vi "ZMQ sandbox.vi"() -> ()   [LabVIEW 2019]
uses:
  <vilib>/addons/zeromq/zmq_context.lvclass
  <vilib>/addons/zeromq/zmq_socket.lvclass
  <vilib>/addons/zeromq/socket_type.ctl
  <vilib>/addons/zeromq/zeromq.lvlib
  <vilib>/addons/_JKI Toolkits/Caraya/classes/Test/Test.lvclass
panel:
  in  "stop":bool
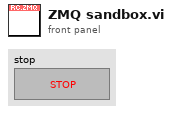
[diagram p1: front panel]
types:
  T1 = typedef "zeromq.lvlib/socket_type.ctl" = enum8{"ZMQ_PAIR", "ZMQ_PUB", "ZMQ_SUB", "ZMQ_REQ", "ZMQ_REP", "ZMQ_DEALER", "ZMQ_ROUTER", "ZMQ_PULL", "ZMQ_PUSH", "ZMQ_XPUB", "ZMQ_XSUB", "ZMQ_STREAM", "ZMQ_SERVER", "ZMQ_CLIENT", "ZMQ_RADIO", "ZMQ_DISH", "ZMQ_GATHER", "ZMQ_SCATTER", "ZMQ_DGRAM"}
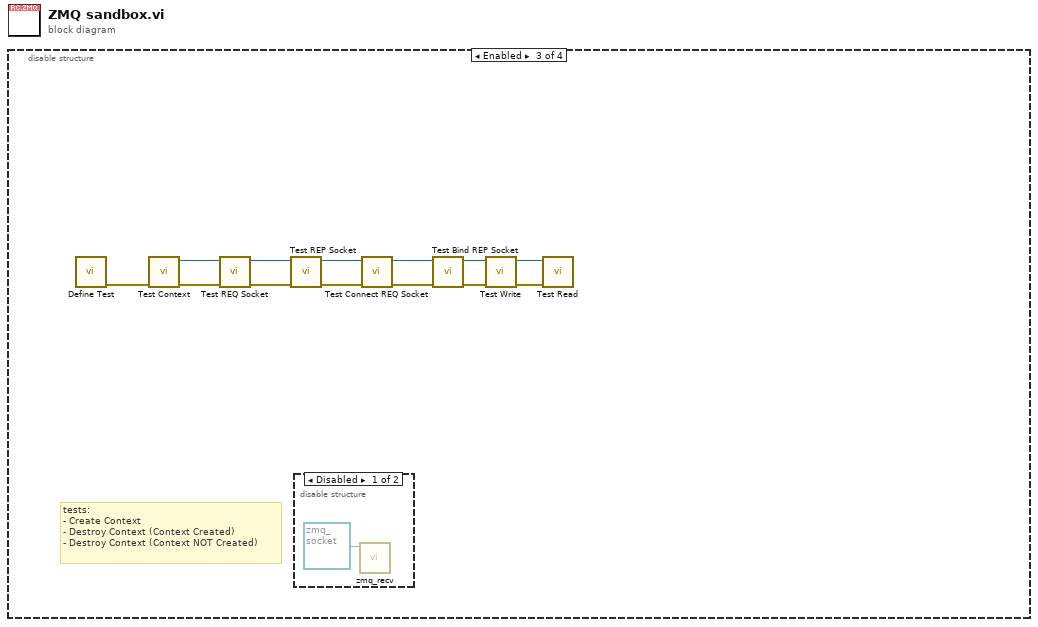
[diagram p0: block diagram]
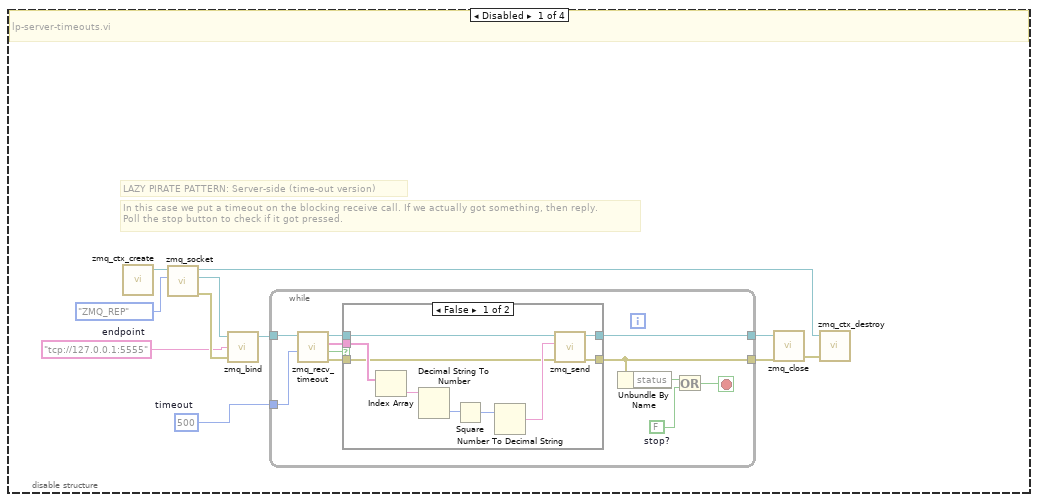
[diagram p2: hidden frame]
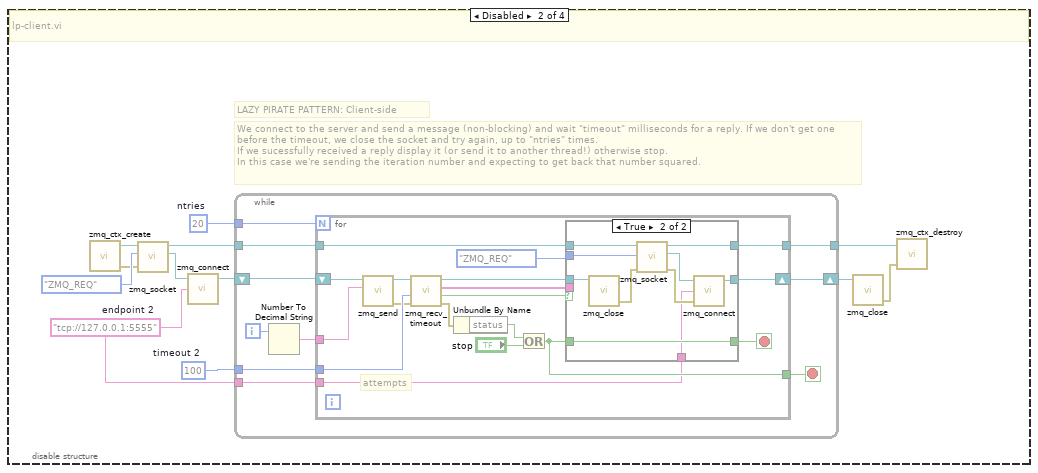
[diagram p4: hidden frame]
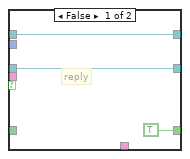
[diagram p5: hidden frame]
diagram:
  n1 = disable-structure "Diagram Disable Structure" shown="Enabled" {
    frame Disabled {
      w11 = u32 500  # timeout
      w9 = "tcp://127.0.0.1:5555"  # endpoint
      # "In this case we put a timeout on the blocking receive call. If we actually got something, then reply.\nPoll the stop button to check if it got pressed."
      # "LAZY PIRATE PATTERN: Server-side (time-out version)"
      # "lp-server-timeouts.vi"
      n2 = call <vilib>:"zmq_ctx_create.vi"() -> ("context out"=w6:refnum<class "zmq_context.lvclass">)  [unwired: 4 in, 1 out]
      n3 = call <vilib>:"zmq_socket.vi"("socket type"=socket_type."ZMQ_REP", "context in"=w6) -> ("error out"=w10:errorcluster, "socket out"=w2:refnum<class "zmq_socket.lvclass">, "context out"=w1:refnum<class "zmq_context.lvclass">)  [unwired: 3 in]
      n4 = call <vilib>:"zmq_bind.vi"("error in"=w10, "endpoint"=w9, "socket in"=w2) -> ("socket out"=w8:refnum<class "zmq_socket.lvclass">)  [unwired: 1 in, 1 out]
      n5 = while {
        tunnel: w11 -> [w20]
        tunnel: w8 -> [w22]
        tunnel: [w17] -> w5
        tunnel: [w16] -> w3
        stop <- w13 stop-if-true
        w14 = FALSE  # stop?
        n6 = call <vilib>:"zmq_recv_timeout.vi"("timeout (ms)"=w20, "socket in"=w22) -> ("error out"=w18:errorcluster, "timeout?"=w12:bool, "parts"=w19:string[], "socket out"=w21:refnum<class "zmq_socket.lvclass">)  [unwired: 2 in]
        n7 = case shown="False" w12 {
          tunnel: w21 -> [w31 w33]
          tunnel: w19 -> [w30 _]
          tunnel: w18 -> [w25 w32]
          tunnel: [w24 w33] -> w17
          tunnel: [w23 w32] -> w16
          frame False {
            n8 = Index Array(array=w30) -> (element=w29:string)  [unwired: 1 in]
            n9 = Decimal String To Number(string=w29) -> (number=w28:i32)  [unwired: 2 in, 1 out]
            n10 = Square(x=w28) -> (x^2=w27:i32)
            n11 = Number To Decimal String(number=w27) -> (decimal integer string=w26:string)  [unwired: 1 in]
            n12 = call <vilib>:"zmq_send.vi"("error in"=w25, "data"=w26, "socket in"=w31) -> ("error out"=w23:errorcluster, "socket out"=w24:refnum<class "zmq_socket.lvclass">)  [unwired: 4 in]
          }
          frame True {
          }
        }
        n13 = Unbundle By Name(w16) -> ("status"=w15:bool)
        n14 = Or(x=w15, y=w14) -> (x .or. y?=w13:bool)
      }
      n15 = call <vilib>:"zmq_close.vi"("error in"=w3, "socket"=w5) -> ("error out"=w4:errorcluster)  [unwired: 3 in]
      n16 = call <vilib>:"zmq_ctx_destroy.vi"("error in"=w4, "context in"=w1) -> ()  [unwired: 3 in, 1 out]
    }
    frame Disabled {
      w34 = "tcp://127.0.0.1:5555"  # endpoint 2
      w45 = u32 100  # timeout 2
      w44 = 20  # ntries
      # "We connect to the server and send a message (non-blocking) and wait \"timeout\" milliseconds for a reply. If we don't get one before the timeout, we close the socket and try again, up to \"ntries\" times.\nIf we sucessfully received a reply display it (or send it to another thread!) otherwise stop.\nIn this case we're sending the iteration number and expecting to get back that number squared."
      # "LAZY PIRATE PATTERN: Client-side"
      # "lp-client.vi"
      n17 = call <vilib>:"zmq_ctx_create.vi"() -> ("error out"=w35:errorcluster, "context out"=w43:refnum<class "zmq_context.lvclass">)  [unwired: 4 in]
      n18 = call <vilib>:"zmq_socket.vi"("error in"=w35, "socket type"=socket_type."ZMQ_REQ", "context in"=w43) -> ("socket out"=w41:refnum<class "zmq_socket.lvclass">, "context out"=w40:refnum<class "zmq_context.lvclass">)  [unwired: 2 in, 1 out]
      n19 = call <vilib>:"zmq_connect.vi"("endpoint"=w34, "socket in"=w41) -> ("socket out"=w39:refnum<class "zmq_socket.lvclass">)  [unwired: 2 in, 1 out]
      n20 = while {
        tunnel: w40 -> [w55]
        tunnel: w45 -> [w54]
        tunnel: w44 -> [w53]
        tunnel: [w48] -> w38
        shift-right: [w47] -> w37
        shift-left: w39 -> [w49]
        tunnel: w34 -> [w46]
        i -> [w52]
        stop <- w50 stop-if-true
        n21 = Number To Decimal String(number=w52) -> (decimal integer string=w51:string)  [unwired: 1 in]
        n22 = for {
          N: w53 -> [_]
          tunnel: w55 -> [w60]
          tunnel: w54 -> [w72]
          tunnel: w51 -> [w68]
          tunnel: [w63] -> w50
          shift-right: [w59] -> w47
          shift-left: w49 -> [w61]
          tunnel: [w58] -> w48
          tunnel: w46 -> [w56]
          stop <- w62 stop-if-true
          # "attempts"
          n23 = call <vilib>:"zmq_send.vi"("data"=w68, "socket in"=w61) -> ("error out"=w69:errorcluster, "socket out"=w70:refnum<class "zmq_socket.lvclass">)  [unwired: 5 in]
          n24 = call <vilib>:"zmq_recv_timeout.vi"("error in"=w69, "timeout (ms)"=w72, "socket in"=w70) -> ("error out"=w67:errorcluster, "timeout?"=w66:bool, "parts"=w71:string[], "socket out"=w73:refnum<class "zmq_socket.lvclass">)  [unwired: 1 in]
          n25 = Unbundle By Name(w67) -> ("status"=w65:bool)
          n26 = Or(x=w65, y="stop") -> (x .or. y?=w63:bool)
          n27 = case shown="True" w66 {
            tunnel: w73 -> [w75 w86]
            tunnel: w71 -> [_ _]
            tunnel: w63 -> [_ w85]
            tunnel: [TRUE w85] -> w62
            tunnel: w60 -> [w74 w84]
            tunnel: [w75 w79] -> w59
            tunnel: [w74 w81] -> w58
            tunnel: socket_type."ZMQ_REQ" ("socket type") -> [_ w78]
            tunnel: w56 -> [_ w77]
            frame False {
              # "reply"
            }
            frame True {
              n28 = call <vilib>:"zmq_close.vi"("socket"=w86) -> ("error out"=w83:errorcluster)  [unwired: 4 in]
              n29 = call <vilib>:"zmq_socket.vi"("error in"=w83, "socket type"=w78, "context in"=w84) -> ("error out"=w82:errorcluster, "socket out"=w80:refnum<class "zmq_socket.lvclass">, "context out"=w81:refnum<class "zmq_context.lvclass">)  [unwired: 2 in]
              n30 = call <vilib>:"zmq_connect.vi"("error in"=w82, "endpoint"=w77, "socket in"=w80) -> ("socket out"=w79:refnum<class "zmq_socket.lvclass">)  [unwired: 1 in, 1 out]
            }
          }
        }
      }
      n31 = call <vilib>:"zmq_close.vi"("socket"=w37) -> ("error out"=w36:errorcluster)  [unwired: 4 in]
      n32 = call <vilib>:"zmq_ctx_destroy.vi"("error in"=w36, "context in"=w38) -> ()  [unwired: 3 in, 1 out]
    }
    frame Enabled {
      # "tests:\n- Create Context\n- Destroy Context (Context Created)\n- Destroy Context (Context NOT Created)"
      n33 = call <vilib>:"Define Test.vi"() -> ("error out"=w99:errorcluster)  [unwired: 10 in, 1 out]
      n34 = call "Test Context.vi"("error in (no error)"=w99) -> ("error out"=w97:errorcluster, "RemoteControl.ZMQ out"=w98:refnum<class "RemoteControl.ZMQ.lvclass">)  [unwired: 9 in]
      n35 = call "Test REQ Socket.vi"("error in (no error)"=w97, "RemoteControl.ZMQ in"=w98) -> ("error out"=w95:errorcluster, "RemoteControl.ZMQ out"=w96:refnum<class "RemoteControl.ZMQ.lvclass">)  [unwired: 8 in]
      n36 = call "Test REP Socket.vi"("error in (no error)"=w95, "RemoteControl.ZMQ in"=w96) -> ("error out"=w93:errorcluster, "RemoteControl.ZMQ out"=w94:refnum<class "RemoteControl.ZMQ.lvclass">)  [unwired: 8 in]
      n37 = disable-structure shown="Disabled" {
        frame Disabled {
          n38 = call <vilib>:"zmq_recv.vi"("socket in"=refnum<class "zmq_socket.lvclass"> refnum) -> ()  [unwired: 4 in, 5 out]
        }
        frame Enabled {
        }
      }
      n39 = call "Test Connect REQ Socket.vi"("error in (no error)"=w93, "RemoteControl.ZMQ in"=w94) -> ("error out"=w91:errorcluster, "RemoteControl.ZMQ out"=w92:refnum<class "RemoteControl.ZMQ.lvclass">)  [unwired: 8 in]
      n40 = call "Test Bind REP Socket.vi"("error in (no error)"=w91, "RemoteControl.ZMQ in"=w92) -> ("error out"=w89:errorcluster, "RemoteControl.ZMQ out"=w90:refnum<class "RemoteControl.ZMQ.lvclass">)  [unwired: 8 in]
      n41 = call "Test Write.vi"("error in (no error)"=w89, "RemoteControl.ZMQ in"=w90) -> ("error out"=w87:errorcluster, "RemoteControl.ZMQ out"=w88:refnum<class "RemoteControl.ZMQ.lvclass">)  [unwired: 8 in]
      n42 = call "Test Read.vi"("error in (no error)"=w87, "RemoteControl.ZMQ in"=w88) -> ()  [unwired: 8 in, 2 out]
    }
    frame Disabled {
    }
  }
